vi "Windows.Lock.vi"(0 "Action":T1(ring), 3 "Show/Enable":bool) -> ()   [LabVIEW 2019, in "Tools.lvlib"]
uses:
  Tools.lvlib
  WinLockDll.dll
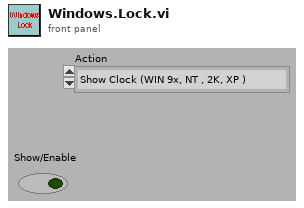
[diagram p1: front panel]
types:
  T1 = enum16{"Show Clock (WIN 9x, NT , 2K, XP )", "Show Taskbar (WIN 9x, NT , 2K, XP )", "Show Start Button (WIN 9x, NT , 2K, XP )", "Show Desktop (WIN 9x, NT , 2K, XP )", "Enable Keys ( Win 9x )", "ALT Tab Enable ( win ? )", "ALT Tab Enable  (WINNT , 2K )", "Enable TaskSwitching  (WINNT , 2K )", "Enable TaskManager (WINNT , 2K )", "Enable CtrlAltDel (WINNT , 2K)"}
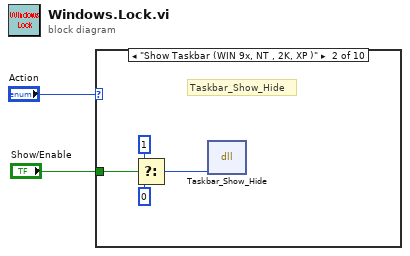
[diagram p0: block diagram]
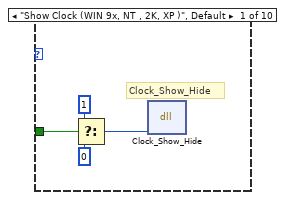
[diagram p2: hidden frame]
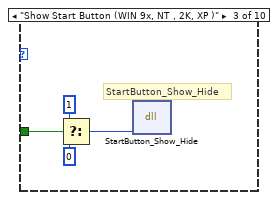
[diagram p3: hidden frame]
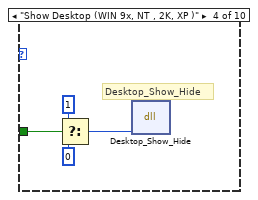
[diagram p4: hidden frame]
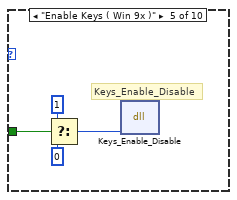
[diagram p5: hidden frame]
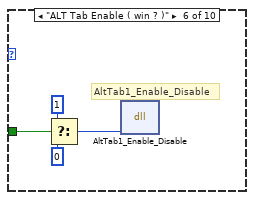
[diagram p6: hidden frame]
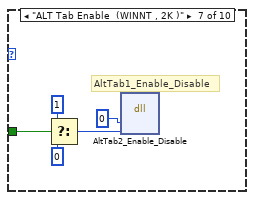
[diagram p7: hidden frame]
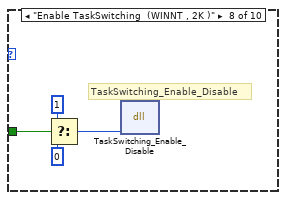
[diagram p8: hidden frame]
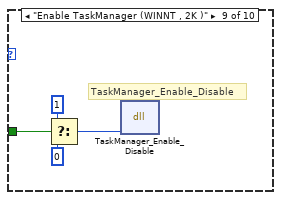
[diagram p9: hidden frame]
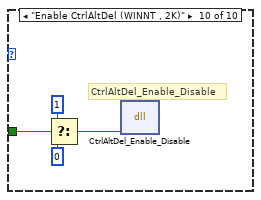
[diagram p10: hidden frame]
diagram:
  n1 = case shown="\"Show Taskbar (WIN 9x, NT , 2K, XP )\"" "Action" {
    tunnel: "Show/Enable" -> [w3 w7 w11 w15 w19 w23 w29 w33 w37 w41]
    frame "Show Clock (WIN 9x, NT , 2K, XP )", Default {
      # "Clock_Show_Hide"
      n2 = Select(t=1, s=w3, f=0) -> (s? t:f=w6:i32)
      n3 = dll-call lib="C:/Projects/_Prywatne/MyCIT/Framework/Tools/Windows/WinLockDll.dll" fn="Clock_Show_Hide"("Show"=w6) -> ()  [unwired: 4 in, 3 out]
    }
    frame "Show Taskbar (WIN 9x, NT , 2K, XP )" {
      # "Taskbar_Show_Hide"
      n4 = Select(t=1, s=w7, f=0) -> (s? t:f=w10:i32)
      n5 = dll-call lib="C:/Projects/_Prywatne/MyCIT/Framework/Tools/Windows/WinLockDll.dll" fn="Taskbar_Show_Hide"("Show"=w10) -> ()  [unwired: 4 in, 3 out]
    }
    frame "Show Start Button (WIN 9x, NT , 2K, XP )" {
      # "StartButton_Show_Hide"
      n6 = Select(t=1, s=w11, f=0) -> (s? t:f=w14:i32)
      n7 = dll-call lib="C:/Projects/_Prywatne/MyCIT/Framework/Tools/Windows/WinLockDll.dll" fn="StartButton_Show_Hide"("Show"=w14) -> ()  [unwired: 4 in, 3 out]
    }
    frame "Show Desktop (WIN 9x, NT , 2K, XP )" {
      # "Desktop_Show_Hide"
      n8 = Select(t=1, s=w15, f=0) -> (s? t:f=w18:i32)
      n9 = dll-call lib="C:/Projects/_Prywatne/MyCIT/Framework/Tools/Windows/WinLockDll.dll" fn="Desktop_Show_Hide"("Show"=w18) -> ()  [unwired: 4 in, 3 out]
    }
    frame "Enable Keys ( Win 9x )" {
      # "Keys_Enable_Disable"
      n10 = Select(t=1, s=w19, f=0) -> (s? t:f=w22:i32)
      n11 = dll-call lib="C:/Projects/_Prywatne/MyCIT/Framework/Tools/Windows/WinLockDll.dll" fn="Keys_Enable_Disable"("Show"=w22) -> ()  [unwired: 4 in, 3 out]
    }
    frame "ALT Tab Enable ( win ? )" {
      # "AltTab1_Enable_Disable"
      n12 = Select(t=1, s=w23, f=0) -> (s? t:f=w26:i32)
      n13 = dll-call lib="C:/Projects/_Prywatne/MyCIT/Framework/Tools/Windows/WinLockDll.dll" fn="AltTab1_Enable_Disable"("Show"=w26) -> ()  [unwired: 4 in, 3 out]
    }
    frame "ALT Tab Enable  (WINNT , 2K )" {
      # "AltTab1_Enable_Disable"
      n14 = Select(t=1, s=w29, f=0) -> (s? t:f=w28:i32)
      n15 = dll-call lib="C:/Projects/_Prywatne/MyCIT/Framework/Tools/Windows/WinLockDll.dll" fn="AltTab2_Enable_Disable"("HWND"=0, "Show"=w28) -> ()  [unwired: 5 in, 3 out]
    }
    frame "Enable TaskSwitching  (WINNT , 2K )" {
      # "TaskSwitching_Enable_Disable"
      n16 = Select(t=1, s=w33, f=0) -> (s? t:f=w32:i32)
      n17 = dll-call lib="C:/Projects/_Prywatne/MyCIT/Framework/Tools/Windows/WinLockDll.dll" fn="TaskSwitching_Enable_Disable"("Show"=w32) -> ()  [unwired: 4 in, 3 out]
    }
    frame "Enable TaskManager (WINNT , 2K )" {
      # "TaskManager_Enable_Disable"
      n18 = Select(t=1, s=w37, f=0) -> (s? t:f=w36:i32)
      n19 = dll-call lib="C:/Projects/_Prywatne/MyCIT/Framework/Tools/Windows/WinLockDll.dll" fn="TaskManager_Enable_Disable"("Show"=w36) -> ()  [unwired: 4 in, 3 out]
    }
    frame "Enable CtrlAltDel (WINNT , 2K)" {
      # "CtrlAltDel_Enable_Disable"
      n20 = Select(t=1, s=w41, f=0) -> (s? t:f=w40:i32)
      n21 = dll-call lib="C:/Projects/_Prywatne/MyCIT/Framework/Tools/Windows/WinLockDll.dll" fn="CtrlAltDel_Enable_Disable"("Show"=w40) -> ()  [unwired: 4 in, 3 out]
    }
  }
